vi "StringToU16(cast).vi"(1 "String":string) -> (0 "U16":u16)   [LabVIEW 2012]
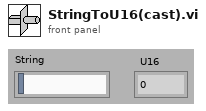
[diagram p1: front panel]
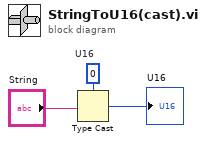
[diagram p0: block diagram]
diagram:
  w2 = u16 0  # U16
  n1 = Type Cast(type=w2, x="String") -> (*(type *) &x=→"U16":u16)
